vi "onCreateDebugTerminal.vi"(8 "error in (no error)":errorcluster, 11 "DebuggingTerminal in":refnum<class "DebuggingTerminal.lvclass">) -> (0 "error out":errorcluster, 3 "DebuggingTerminal out":refnum<class "DebuggingTerminal.lvclass">)   [LabVIEW 2013, in "MQTT Base.lvlib" / "DebuggingTerminal.lvclass"]
uses:
  DebuggingTerminal.lvclass
  DebuggingTerminal.lvclass/DebuggingTerminal.ctl
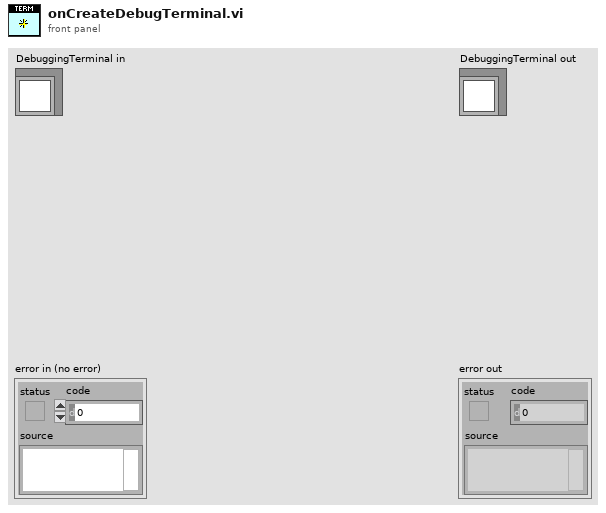
[diagram p1: front panel]
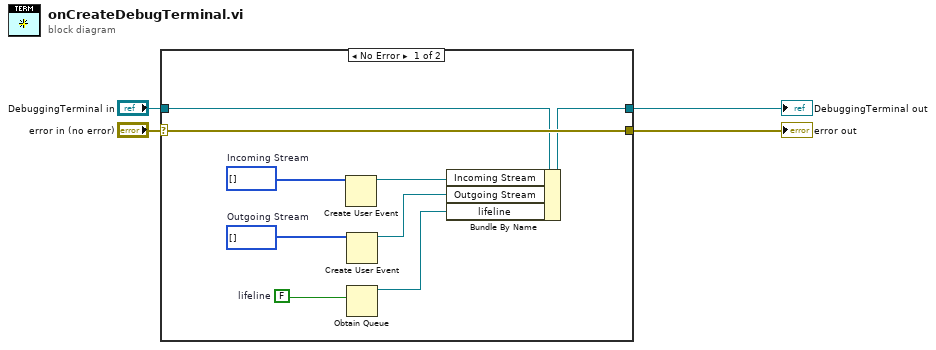
[diagram p0: block diagram]
diagram:
  n1 = case shown="No Error" "error in (no error)" {
    selector: "error in (no error)" -> [w13 w15]
    tunnel: [w13 w15] -> w3
    tunnel: [w7 w14] -> w1
    tunnel: "DebuggingTerminal in" -> [w12 w14]
    frame No Error {
      w6 = FALSE  # lifeline
      w10 = u8[] []  # Outgoing Stream
      w11 = u8[] []  # Incoming Stream
      n2 = Create User Event(user event datatype=w11) -> (user event=w9:refnum<user-event>)  [unwired: 1 in, 1 out]
      n3 = Create User Event(user event datatype=w10) -> (user event=w8:refnum<user-event>)  [unwired: 1 in, 1 out]
      n4 = Obtain Queue(element data type=w6) -> (queue out=w5:refnum<queue>)  [unwired: 4 in, 2 out]
      n5 = Bundle By Name(cluster=w12, "Incoming Stream"=w9, "Outgoing Stream"=w8, "lifeline"=w5) -> (w7:refnum<class "DebuggingTerminal.lvclass">)
    }
    frame Error {
    }
  }
  "error out" <- w3
  "DebuggingTerminal out" <- w1
